vi "Add Key-Value Pair.vi"(7 "overwrite?":bool=TRUE, 9 "error in (no error)":errorcluster, 10 "entry":cluster{"key":string, "value":variant}, 11 "Properties in":refnum<class "Properties.lvclass">) -> (1 "error out":errorcluster, 3 "Properties out":refnum<class "Properties.lvclass">)   [LabVIEW 2020, in "Caraya.lvlib" / "Properties.lvclass"]
uses:
  Properties.lvclass
  Properties.lvclass/Properties.ctl
  Test Manager Message KVP/TestManagerMsg.KVP.lvclass
  Caraya.lvlib
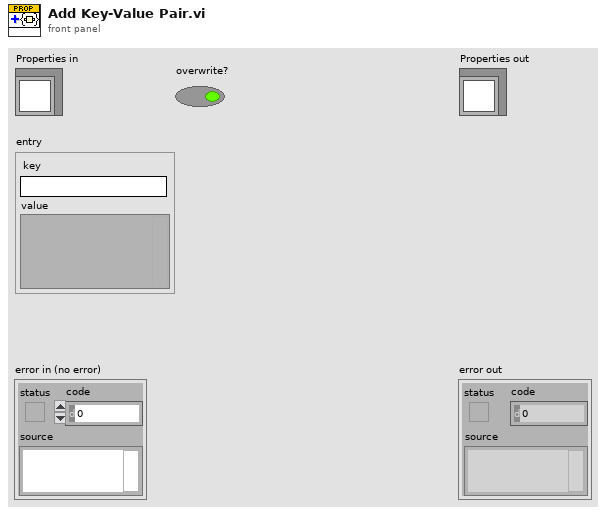
[diagram p1: front panel]
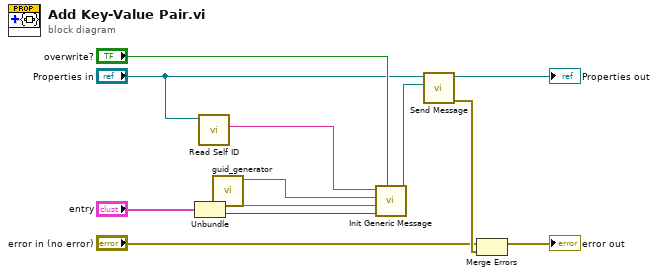
[diagram p0: block diagram]
diagram:
  n1 = Unbundle("entry") -> ("key"=w9:string, "value"=w8:variant)
  n2 = call "Read Self ID.vi"("Properties in"="Properties in") -> ("self-id"=w2:string)  [unwired: 9 in, 1 out]
  n3 = call "guid_generator.vi"() -> ("guid"=w1:string)  [unwired: 11 in]
  n4 = call "Init Generic Message.vi"("overwrite?"="overwrite?", "value"=w8, "key"=w9, "self-id"=w1, "owner-id"=w2) -> ("Message"=w7:refnum<class "TestManagerMsg.lvclass">)  [unwired: 6 in]
  n5 = call "Send Message.vi"("TestManagerMsg"=w7, "Properties in"="Properties in") -> ("error out"=w4:errorcluster, "Properties out"=→"Properties out":refnum<class "Properties.lvclass">)  [unwired: 8 in]
  n6 = Merge Errors("error in (no error)", w4) -> (→"error out":errorcluster)
